vi "Average Image Color.vi"(11 "Refnum in":T1) -> (0 "B":dbl, 1 "G":dbl, 2 "R":dbl, 3 "Refnum out":T1)   [LabVIEW 2014]
uses:
  <vilib>/vision/Image Controls.llb/IMAQ Image.ctl
  <vilib>/vision/NI_Vision_Development_Module.lvlib
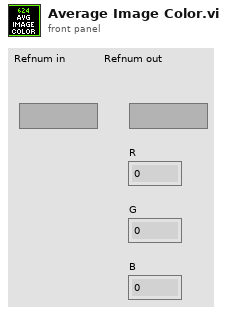
[diagram p1: front panel]
types:
  T1 = typedef "IMAQ Image.ctl" = refnum<image>
  T2 = typedef "Image Type" = u32
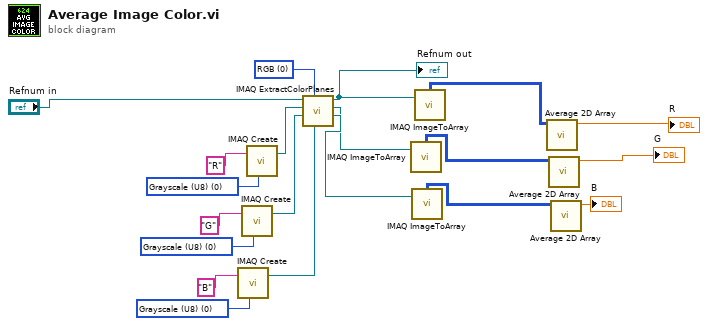
[diagram p0: block diagram]
diagram:
  w9 = T2 0 items=["Grayscale (U8)", "Grayscale (I16)", "Grayscale (SGL)", "Complex (CSG)", "RGB (U32)", "HSL (U32)", "RGB (U64)", "Grayscale (U16)"] ("Image Type")
  w7 = T2 0 items=["Grayscale (U8)", "Grayscale (I16)", "Grayscale (SGL)", "Complex (CSG)", "RGB (U32)", "HSL (U32)", "RGB (U64)", "Grayscale (U16)"] ("Image Type")
  w3 = T2 0 items=["Grayscale (U8)", "Grayscale (I16)", "Grayscale (SGL)", "Complex (CSG)", "RGB (U32)", "HSL (U32)", "RGB (U64)", "Grayscale (U16)"] ("Image Type")
  w2 = u16 0 items=["RGB", "HSL", "HSV", "HSI"] ("Color Mode")
  n1 = call "IMAQ Create"("Image Name"="B", "Image Type"=w9) -> ("New Image"=w11:T1)  [unwired: 3 in, 1 out]
  n2 = call "IMAQ Create"("Image Name"="G", "Image Type"=w7) -> ("New Image"=w8:T1)  [unwired: 3 in, 1 out]
  n3 = call "IMAQ Create"("Image Name"="R", "Image Type"=w3) -> ("New Image"=w5:T1)  [unwired: 3 in, 1 out]
  n4 = call "IMAQ ExtractColorPlanes"("Blue or Luma or Val or Inten Plane"=w11, "Color Mode"=w2, "Green or Sat Plane"=w8, "Red or Hue Plane"=w5, "Image Src"="Refnum in") -> ("Blue or Luma or Val or Inten Plane out"=w16:T1, "Green or Sat Plane out"=w15:T1, "Red or Hue Plane out"=w12:T1)  [unwired: 3 in, 1 out]
  "Refnum out" <- w12
  n5 = call "IMAQ ImageToArray"("Image"=w15) -> ("Image Pixels (U8)"=w17:u8[][])  [unwired: 3 in, 4 out]
  n6 = call "IMAQ ImageToArray"("Image"=w16) -> ("Image Pixels (U8)"=w18:u8[][])  [unwired: 3 in, 4 out]
  n7 = call "IMAQ ImageToArray"("Image"=w12) -> ("Image Pixels (U8)"=w13:u8[][])  [unwired: 3 in, 4 out]
  n8 = call "Average 2D Array.vi"("Image Pixels (U8)"=w13) -> ("Numeric"=→"R":dbl)  [unwired: 10 in]
  n9 = call "Average 2D Array.vi"("Image Pixels (U8)"=w17) -> ("Numeric"=→"G":dbl)  [unwired: 10 in]
  n10 = call "Average 2D Array.vi"("Image Pixels (U8)"=w18) -> ("Numeric"=→"B":dbl)  [unwired: 10 in]
